vi "From String Array.vi"(8 "error in (no error)":errorcluster, 9 "String Array":string[](array[string]), 11 "Conditional Jump Step Config in":refnum<class "Conditional Jump Step Config.lvclass">) -> (0 "error out":errorcluster, 1 "String Array 2":string[](array[string]), 3 "Conditional Jump Step Config out":refnum<class "Conditional Jump Step Config.lvclass">)   [LabVIEW 2015, in "Conditional Jump Step Config.lvclass"]
uses:
  Conditional Jump Step Config.lvclass
  <vilib>/NI/Tag Bus Module Framework/channel/TBM channel.lvclass
  <vilib>/NI/Tag Bus/tag/Data Type.ctl
  <vilib>/NI/Tag Bus/tag/tag descriptor.lvclass
  <vilib>/NI/Tag Bus Module Framework/channel/channel classification.ctl
  classes/Step/Config/Step Config.lvclass
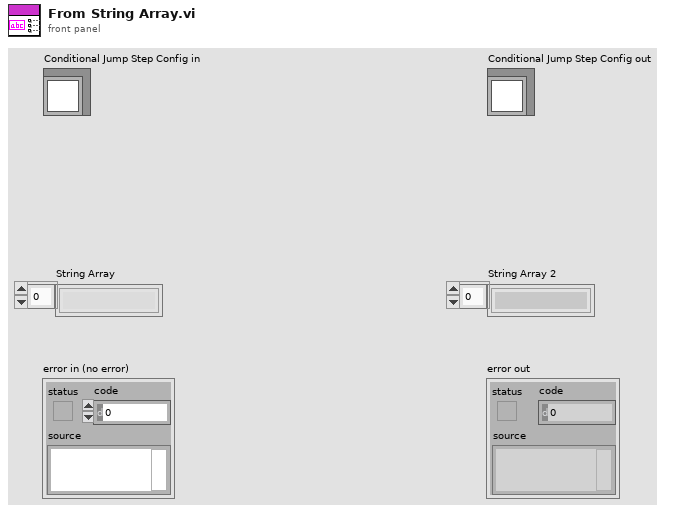
[diagram p1: front panel]
types:
  T1 = typedef "TBM channel.lvclass/channel classification.ctl" = enum16{"input data", "output data", "processing parameter", "processing result"}
  T2 = typedef "tag bus.lvlib/tag descriptor.lvclass/Data Type.ctl" = enum16{"Double", "Single", "I64", "I32", "I16", "I8", "U64", "U32", "U16", "U8", "Boolean", "String", "Array of Double", "Array of Single", "Array of I64", "Array of I32", "Array of I16", "Array of I8", "Array of U64", "Array of U32", "Array of U16", "Array of U8", "Array of Boolean", "Array of String"}
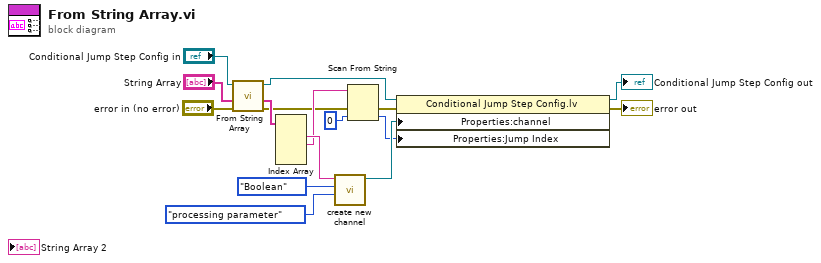
[diagram p0: block diagram]
diagram:
  n1 = call-parent "From String Array.vi"("error in (no error)"="error in (no error)", "String Array"="String Array", "Step Config in"="Conditional Jump Step Config in") -> ("error out"=w1:errorcluster, "Elements Left 2"=w3:string[], "Step Config out"=w5:refnum<class "Conditional Jump Step Config.lvclass">)  [unwired: 6 in]
  n2 = Index Array(array=w3) -> (element #1=w15:string, element #2=w10:string)  [unwired: 4 in, 2 out]
  n3 = call <vilib>:"create new channel.vi"("channel classification"=channel_classification."processing parameter", "data type"=Data_Type."Boolean", "channel name"=w15) -> ("channel"=w16:refnum<class "TBM channel.lvclass">)  [unwired: 8 in]
  n4 = Scan From String(input string=w10, error in=w1, default 1=0 ("Jump Index")) -> (error out=w7:errorcluster, output 1=w9:i32)  [unwired: 2 in, 2 out]
  n5 = property class="Conditional Jump Step Config.lv"(reference=w5, error in=w7, "Properties:channel"=w16, "Properties:Jump Index"=w9) -> (reference out=→"Conditional Jump Step Config out":refnum<class "Conditional Jump Step Config.lvclass">, error out=→"error out":errorcluster)
